vi "h5_write_1d_double_array.vi"(0 "h5 ref in":i32, 1 "dataset name":string, 5 "array":dbl[](array[numeric]), 7 "units (au)":string="au", 11 "error in (no error)":errorcluster, 12 "dim (index)":string="index") -> (4 "h5 ref out":i32, 15 "error out":errorcluster)   [LabVIEW 2015]
uses:
  <userlib>/_OpenG.lib/string/string.llb/To Camel Case (String)__ogtk.vi
  <vilib>/addons/h5labview2/base/lib_path.vi
  <vilib>/addons/h5labview2/base/H5Equery.vi
  <vilib>/addons/h5labview2/dataset/H5Dwrite.llb/H5Dwrite.xnode
  <vilib>/addons/h5labview2/attrib/H5Awrite.llb/H5Awrite.xnode
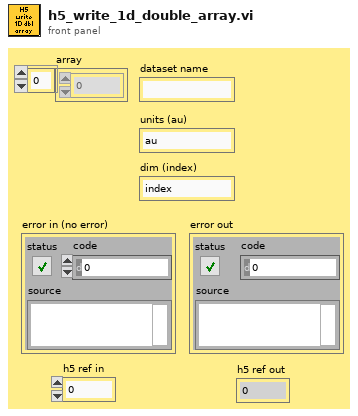
[diagram p1: front panel]
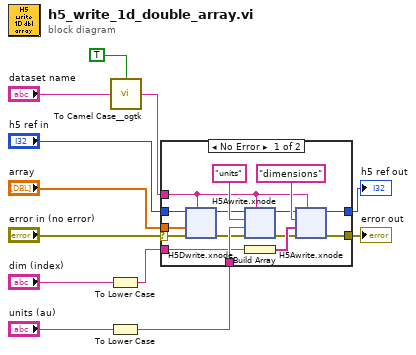
[diagram p0: block diagram]
diagram:
  n1 = To Lower Case(string="dim (index)") -> (all lower case string=w4:string)
  n2 = To Lower Case(string="units (au)") -> (all lower case string=w6:string)
  n3 = call-poly <userlib>:"To Camel Case__ogtk.vi"("string"="dataset name", "no change if no spaces? (F=No)"=TRUE) -> ("CamelCase string"=w2:string)
  n4 = case shown="No Error" "error in (no error)" {
    selector: "error in (no error)" -> [w13 w86]
    tunnel: "h5 ref in" -> [w27 w85]
    tunnel: w6 -> [w25 _]
    tunnel: w4 -> [w23 _]
    tunnel: "array" -> [w21 _]
    tunnel: w2 -> [w16 _]
    tunnel: [w15 w86] -> w10
    tunnel: [w14 w85] -> w9
    frame No Error {
      n5 = xnode "H5Dwrite.xnode"("dataset name"=w16, "error in (no error)"=w13, "data"=w21, "ref in"=w27) -> ("error out"=w20:errorcluster, "ref out"=w18:i32)  [unwired: 3 in, 1 out]
      n6 = xnode "H5Awrite.xnode"("object name"=w16, "error in (no error)"=w20, "data"=w25, "attrib name"="units", "ref in"=w18) -> ("error out"=w19:errorcluster, "ref out"=w17:i32)  [unwired: 2 in, 1 out]
      n7 = Build Array(w23) -> (w22:string[])
      n8 = xnode "H5Awrite.xnode"("object name"=w16, "error in (no error)"=w19, "data"=w22, "attrib name"="dimensions", "ref in"=w17) -> ("error out"=w15:errorcluster, "ref out"=w14:i32)  [unwired: 2 in, 1 out]
    }
    frame Error {
    }
  }
  "error out" <- w10
  "h5 ref out" <- w9
